vi "WM Output Settings.vi"(1 "Output Settings":T2={"Device"=1, "Channel"="0", "Sampling Rate"=200, "Ramp Time"=2.0, "Buffer Length"=4, "Buffer Size"=65536, "Sub Buffer Length"=1, "Sub Buffer Size"=128} {"Ramp Time" min=0.0 format="%.2f"; "Sub Buffer Length" items=["0 : 0.3", "0 : 0.6", "0 : 1.3", "0 : 2.6", "0 : 5.1", "0 : 10.2"]; "Buffer Length" items=["  0 : 20.5", "  0 : 41.0", "  1 : 21.9", "  2 : 43.8", "  5 : 27.7", " 10 : 55.4", " 21 : 50.7"]; "Sampling Rate" min=1}) -> (0 "Output Settings Results":T1={"Device"=1, "Channel"="0", "Sampling Rate"=200, "Stroke Calibration"=0.0, "Buffer Length"=4, "Buffer Size"=0, "Sub Buffer Length"=1, "Sub Buffer Size"=0} {"Stroke Calibration" format="%.2f"; "Sub Buffer Length" items=["0 : 0.3", "0 : 0.6", "0 : 1.3", "0 : 2.6", "0 : 5.1", "0 : 10.2"]; "Buffer Length" items=["  0 : 20.5", "  0 : 41.0", "  1 : 21.9", "  2 : 43.8", "  5 : 27.7", " 10 : 55.4", " 21 : 50.7"]; "Sampling Rate" min=1})   [LabVIEW 2012]
panel:
  in  "OK":bool
  # "min:sec"
  # "Hz"
  # "min:sec"
  # "V/m"
  # "min:sec"
  # "Hz"
  # "min:sec"
  # "s"
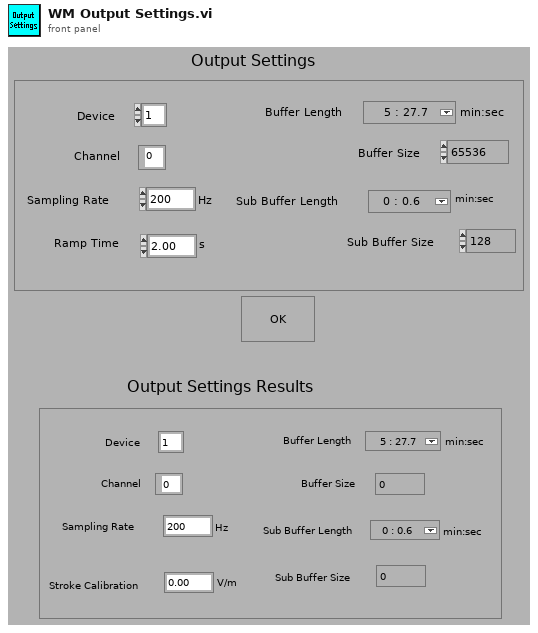
[diagram p1: front panel]
types:
  T1 = cluster{"Device":i16, "Channel":string, "Sampling Rate":i32, "Stroke Calibration":dbl, "Buffer Length":u16, "Buffer Size":i32, "Sub Buffer Length":i16, "Sub Buffer Size":i16}
  T2 = cluster{"Device":i16, "Channel":string, "Sampling Rate":i32, "Ramp Time":dbl, "Buffer Length":u16, "Buffer Size":i32, "Sub Buffer Length":i16, "Sub Buffer Size":i16}
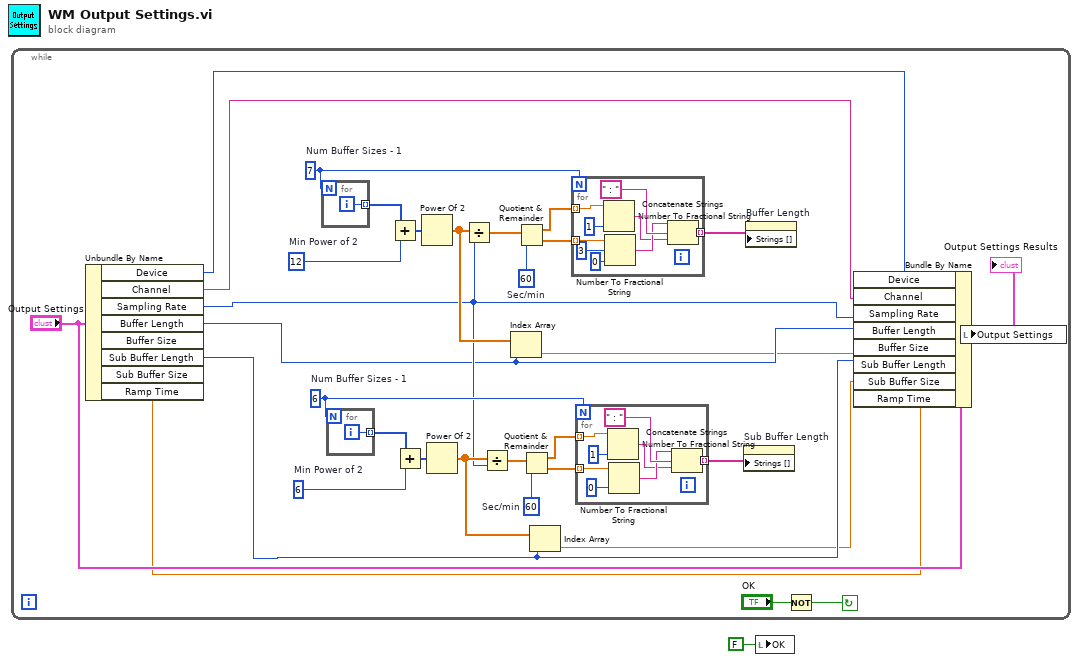
[diagram p0: block diagram]
diagram:
  n1 = while {
    stop <- w3 continue-if-true
    w21 = 60  # Sec/min
    w24 = 6  # Min Power of 2
    w18 = 6  # Num Buffer Sizes - 1
    w30 = 60  # Sec/min
    w33 = 12  # Min Power of 2
    w27 = 7  # Num Buffer Sizes - 1
    n2 = Unbundle By Name("Output Settings") -> ("Device"=w12:i16, "Channel"=w11:string, "Sampling Rate"=w10:i32, "Buffer Length"=w9:u16, "Sub Buffer Length"=w7:i16, "Ramp Time"=w2:dbl)  [unwired: 2 out]
    n3 = for {
      N: w27 -> [_]
      tunnel: [w52] -> w32 mode=indexing
      i -> [w52]
    }
    n4 = for {
      N: w18 -> [_]
      tunnel: [w42] -> w23 mode=indexing
      i -> [w42]
    }
    n5 = Add(x=w32, y=w33) -> (x+y=w31:i32[])
    n6 = Add(x=w23, y=w24) -> (x+y=w22:i32[])
    n7 = Power Of 2(x=w31) -> (2^x=w25:dbl[])
    n8 = Power Of 2(x=w22) -> (2^x=w16:dbl[])
    n9 = Divide(x=w25, y=w10) -> (x/y=w26:dbl[])
    n10 = Divide(x=w16, y=w10) -> (x/y=w17:dbl[])
    n11 = Index Array(array=w25, index=w9) -> (element=w8:dbl)
    n12 = Quotient & Remainder(x=w26, y=w30) -> (x-y*floor(x/y)=w28:dbl[], floor(x/y)=w29:dbl[])
    n13 = Quotient & Remainder(x=w17, y=w21) -> (x-y*floor(x/y)=w19:dbl[], floor(x/y)=w20:dbl[])
    n14 = Index Array(array=w16, index=w7) -> (element=w6:dbl)
    n15 = for {
      N: w27 -> [_]
      tunnel: w29 -> [w51] mode=indexing
      tunnel: w28 -> [w50] mode=indexing
      tunnel: [w48] -> w15 mode=indexing
      n16 = Number To Fractional String(number=w50, precision (6)=i16 1) -> (F-format string=w46:string)  [unwired: 2 in]
      n17 = Number To Fractional String(number=w51, width (-)=i16 3, precision (6)=i16 0 ("width (-)")) -> (F-format string=w47:string)  [unwired: 1 in]
      n18 = Concatenate Strings(w47, " : " ("Substring"), w46) -> (w48:string)
    }
    n19 = for {
      N: w18 -> [_]
      tunnel: w20 -> [w41] mode=indexing
      tunnel: w19 -> [w40] mode=indexing
      tunnel: [w38] -> w14 mode=indexing
      n20 = Number To Fractional String(number=w40, precision (6)=i16 1) -> (F-format string=w36:string)  [unwired: 2 in]
      n21 = Number To Fractional String(number=w41, precision (6)=i16 0 ("width (-)")) -> (F-format string=w37:string)  [unwired: 2 in]
      n22 = Concatenate Strings(w37, " : " ("Substring"), w36) -> (w38:string)
    }
    n23 = property on="Sub Buffer Length" class="Ring (strict)"("Strings []"=w14) -> ()  [unwired: 2 in, 2 out]
    n24 = property on="Buffer Length" class="Ring (strict)"("Strings []"=w15) -> ()  [unwired: 2 in, 2 out]
    n25 = Not(x="OK") -> (.not. x?=w3:bool)
    n26 = Bundle By Name(cluster="Output Settings", "Device"=w12, "Channel"=w11, "Sampling Rate"=w10, "Buffer Length"=w9, "Buffer Size"=w8, "Sub Buffer Length"=w7, "Sub Buffer Size"=w6, "Ramp Time"=w2) -> (w4:T2)
    "Output Settings Results" <- w4
    n27 = local write "Output Settings"(w4) -> ()
  }
  n28 = local write "OK"(FALSE ("OK")) -> ()
